vi "Operation.vi"(0 "Arithmetic_Operations in":refnum<class "Arithmetic_Operations.lvclass">, 11 "Error In":errorcluster) -> (4 "Arithmetic_Operations out":refnum<class "Arithmetic_Operations.lvclass">, 15 "Error Out":errorcluster)   [LabVIEW 2020, in "Arithmetic_Operations.lvclass"]
doc: "This VI is used to over ridden by the child classes."
uses:
  Arithmetic_Operations.lvclass
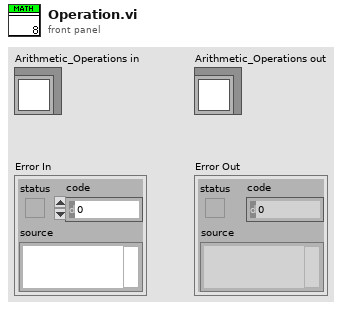
[diagram p1: front panel]
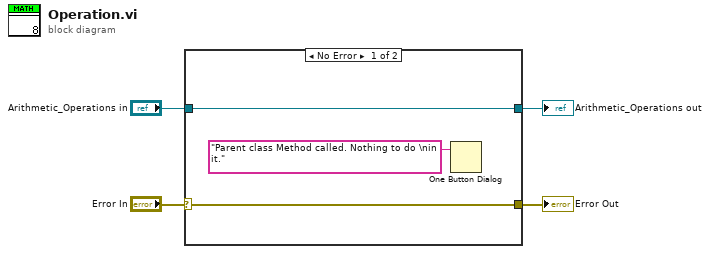
[diagram p0: block diagram]
diagram:
  n1 = case shown="No Error" "Error In" {
    selector: "Error In" -> [w6 w9]
    tunnel: [w6 w9] -> w3
    tunnel: [w7 w8] -> w1
    tunnel: "Arithmetic_Operations in" -> [w7 w8]
    frame No Error {
      n2 = One Button Dialog(message="Parent class Method called. Nothing to do \nin it.") -> ()  [unwired: 1 in, 1 out]
    }
    frame Error {
    }
  }
  "Error Out" <- w3
  "Arithmetic_Operations out" <- w1
